vi "in_diff and divided diff (dy).vi"(11 "Y":dbl[](array[numeric]), 12 "i1":i32, 13 "i2":i32=-1) -> (10 "difference":dbl)   [LabVIEW 2020, in "NI_Gmath.lvlib"]
uses:
  <vilib>/gmath/NI_Gmath.lvlib
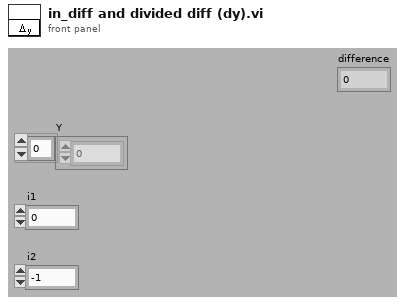
[diagram p1: front panel]
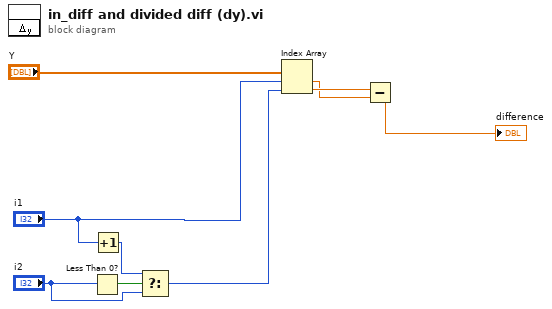
[diagram p0: block diagram]
diagram:
  n1 = Less Than 0?(x="i2") -> (x < 0?=w7:bool)
  n2 = Increment(x="i1") -> (x+1=w4:i32)
  n3 = Select(t=w4, s=w7, f="i2") -> (s? t:f=w3:i32)
  n4 = Index Array(array="Y", index #1="i1", index #2=w3) -> (element #1=w1:dbl, element #2=w2:dbl)
  n5 = Subtract(x=w2, y=w1) -> (x-y=→"difference":dbl)
